vi "Set Team Index.vi"(8 "error in (no error)":errorcluster, 10 "Team Index":i32, 11 "Square in":refnum<class "Square.lvclass">) -> (0 "error out":errorcluster, 3 "Square out":refnum<class "Square.lvclass">)   [LabVIEW 2020, in "SquareBattle.lvlib" / "Square.lvclass"]
uses:
  Square.lvclass
  Square.lvclass/Square.ctl
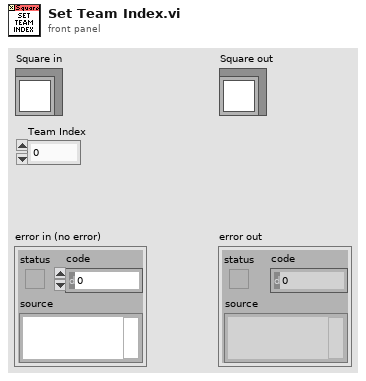
[diagram p1: front panel]
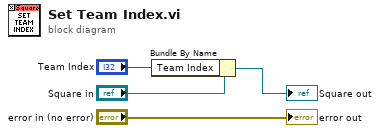
[diagram p0: block diagram]
diagram:
  n1 = Bundle By Name(cluster="Square in", "Team Index"="Team Index") -> (→"Square out":refnum<class "Square.lvclass">)
  "error out" <- "error in (no error)"
